vi "Setup.vi"(8 "error in (no error)":errorcluster, 11 "Assigned VISA Ports":T1(array[cluster])) -> (0 "error out":errorcluster)   [LabVIEW 2018]
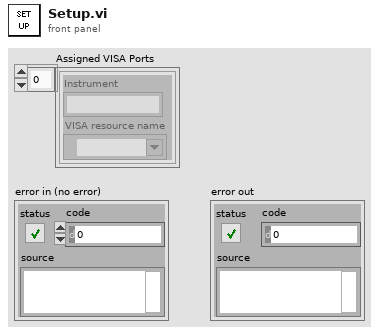
[diagram p1: front panel]
types:
  T1 = cluster{"Instrument":string, "VISA resource name":refnum<visa-resource-name>}[]
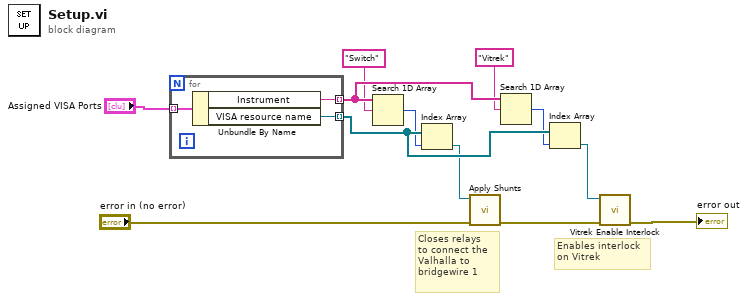
[diagram p0: block diagram]
diagram:
  # "Enables interlock \non Vitrek"
  # "Closes relays\nto connect the \nValhalla to \nbridgewire 1"
  n1 = for {
    tunnel: [w15] -> w8 mode=indexing
    tunnel: [w14] -> w9 mode=indexing
    tunnel: "Assigned VISA Ports" -> [w13] mode=indexing
    n2 = Unbundle By Name(w13) -> ("Instrument"=w15:string, "VISA resource name"=w14:refnum<visa-resource-name>)
  }
  n3 = Search 1D Array(1D array=w8, element="Switch") -> (index of element=w2:i32)  [unwired: 1 in]
  n4 = Index Array(array=w9, index=w2) -> (element=w4:refnum<visa-resource-name>)
  n5 = call "Apply Shunts.vi"("error in (no error)"="error in (no error)", "VISA Refnum in"=w4) -> ("error out"=w5:errorcluster)  [unwired: 9 in]
  n6 = Search 1D Array(1D array=w8, element="Vitrek") -> (index of element=w6:i32)  [unwired: 1 in]
  n7 = Index Array(array=w9, index=w6) -> (element=w10:refnum<visa-resource-name>)
  n8 = call "Vitrek Enable Interlock.vi"("error in (no error)"=w5, "VISA resource name in"=w10) -> ("error out"=→"error out":errorcluster)  [unwired: 9 in]
